vi "Set Pulse Timing.vi"(7 "Output pulse channel":T1, 8 "error in (no error)":errorcluster, 9 "Duration":dbl format="%#_6ps", 10 "Start delay":dbl format="%#_6ps", 11 "Delay Generator Driver in":refnum<class "Delay Generator Driver.lvclass">) -> (0 "error out":errorcluster, 3 "Delay Generator Driver out":refnum<class "Delay Generator Driver.lvclass">)   [LabVIEW 2020, in "Delay Generator Driver.lvclass"]
uses:
  Delay Generator Driver.lvclass
  DG Pulse Output Channel.ctl
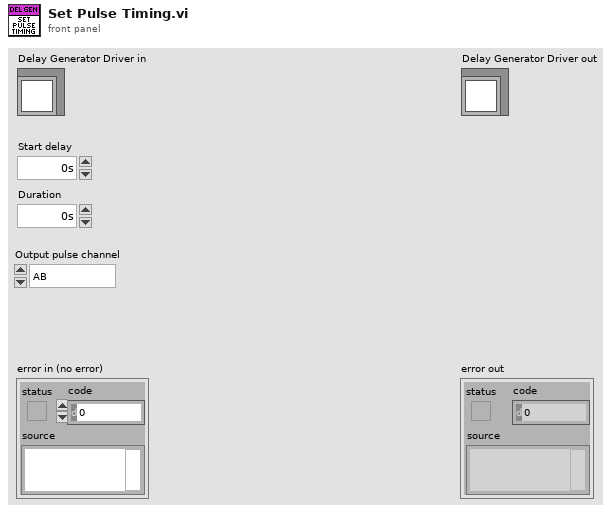
[diagram p1: front panel]
types:
  T1 = typedef "DG Pulse Output Channel.ctl" = enum16{"AB", "CD"}
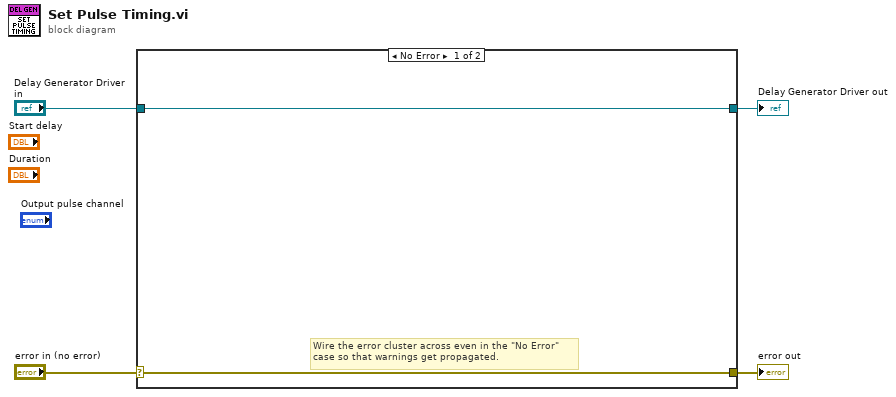
[diagram p0: block diagram]
diagram:
  n1 = case shown="No Error" "error in (no error)" {
    selector: "error in (no error)" -> [w5 w8]
    tunnel: [w5 w8] -> w3
    tunnel: [w6 w7] -> w1
    tunnel: "Delay Generator Driver in" -> [w6 w7]
    frame No Error {
      # "Wire the error cluster across even in the \"No Error\"\ncase so that warnings get propagated."
    }
    frame Error {
    }
  }
  "error out" <- w3
  "Delay Generator Driver out" <- w1
